vi "PH_ImageStatistician.handle Data.vi"(6 "New Img Op Dataset":T1, 7 "Dataarray Size in":i32, 8 "Data in":T1[](array[typedef]), 9 "Datasets strored in":i32) -> (1 "Dataarray Size out":i32, 2 "Data out":T1[](array[typedef]), 3 "Datasets strored out":i32)   [LabVIEW 2014, in "PH_ImageStatistician.lvlib"]
doc: "This VI handles the array made out of new dataset coming in: It creates an array of 3600 enries (values NaN) and replaces them peu a peu by the new incoming dataset. If the array is full, additional 3600 NaN-entries are added and so on ..."
uses:
  PH_ImageStatistician.Statistician Data.ctl
  PH_ImageStatistician.lvlib
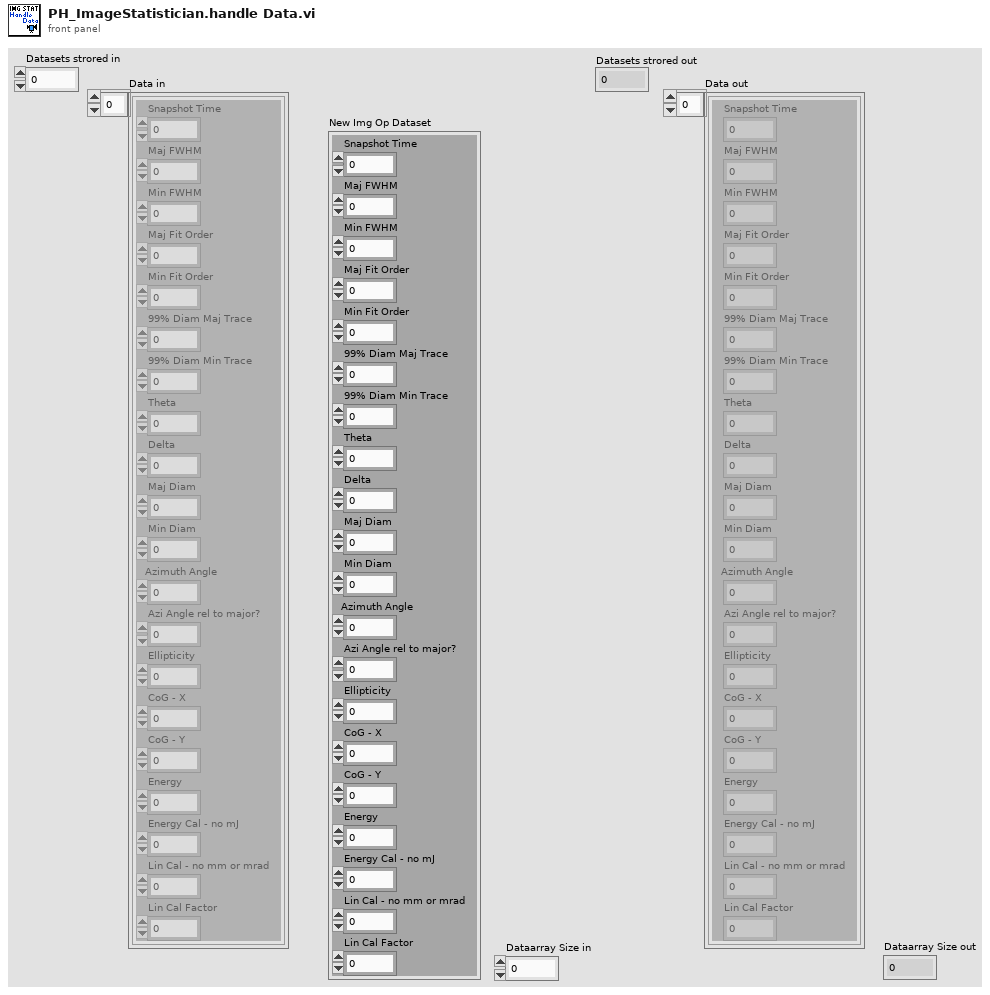
[diagram p1: front panel]
types:
  T1 = typedef "PH_ImageStatistician.lvlib/PH_ImageStatistician.Statistician Data.ctl" = cluster{"Snapshot Time":dbl, "Maj FWHM":dbl, "Min FWHM":dbl, "Maj Fit Order":dbl, "Min Fit Order":dbl, "99% Diam Maj Trace":dbl, "99% Diam Min Trace":dbl, "Theta":dbl, "Delta":dbl, "Maj Diam":dbl, "Min Diam":dbl, "Azimuth Angle":dbl, "Azi Angle rel to major?":dbl, "Ellipticity":dbl, "CoG - X":dbl, "CoG - Y":dbl, "Energy":dbl, "Energy Cal - no mJ":dbl, "Lin Cal - no mm or mrad":dbl, "Lin Cal Factor":dbl}
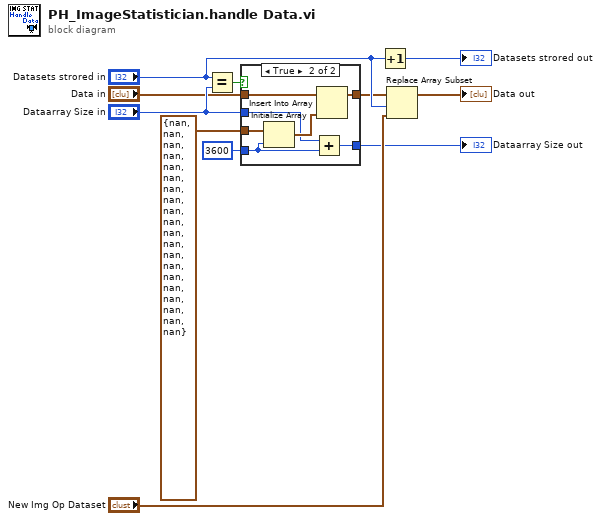
[diagram p0: block diagram]
diagram:
  n1 = Equal?(x="Datasets strored in", y="Dataarray Size in") -> (x = y?=w11:bool)
  n2 = case shown="True" w11 {
    tunnel: "Data in" -> [w13 w20]
    tunnel: [w13 w19] -> w8
    tunnel: "Dataarray Size in" -> [w12 w17]
    tunnel: [w12 w16] -> w4
    tunnel: T1 {"Snapshot Time"=nan, "Maj FWHM"=nan, "Min FWHM"=nan, "Maj Fit Order"=nan, "Min Fit Order"=nan, "99% Diam Maj Trace"=nan, "99% Diam Min Trace"=nan, "Theta"=nan, "Delta"=nan, "Maj Diam"=nan, "Min Diam"=nan, "Azimuth Angle"=nan, "Azi Angle rel to major?"=nan, "Ellipticity"=nan, "CoG - X"=nan, "CoG - Y"=nan, "Energy"=nan, "Energy Cal - no mJ"=nan, "Lin Cal - no mm or mrad"=nan, "Lin Cal Factor"=nan} ("Starter 2") -> [_ w15]
    tunnel: 3600 ("dimension size") -> [_ w14]
    frame False {
    }
    frame True {
      n3 = Initialize Array(w15, w14) -> (w18:T1[])
      n4 = Add(x=w17, y=w14) -> (x+y=w16:i32)
      n5 = Insert Into Array(array=w20, new element=w18) -> (w19:T1[])  [unwired: 1 in]
    }
  }
  "Dataarray Size out" <- w4
  n6 = Increment(x="Datasets strored in") -> (x+1=→"Datasets strored out":i32)
  n7 = Replace Array Subset(array=w8, new element="New Img Op Dataset", index="Datasets strored in") -> (→"Data out":T1[])
